vi "Pfeiffer Vacuum HiLobe Status requests.vi"(8 "error in (no error)":errorcluster, 9 "Parameter choice":T1(ring), 10 "Adress of unit":u16=1 min=1 max=999 step=1, 11 "COM Port Name in":refnum<visa-resource-name>="COM1") -> (0 "error out":errorcluster, 3 "response (data)":string)   [LabVIEW 2021]
doc: "This VI is an example of how to use the Pfeiffer Vacuum subVIs programmatically. This VI first initializes the instrument, takes measurements, then closes the instrument."
uses:
  <instrlib>/Pfeiffer Vacuum/Pfeiffer Vacuum.lvlib
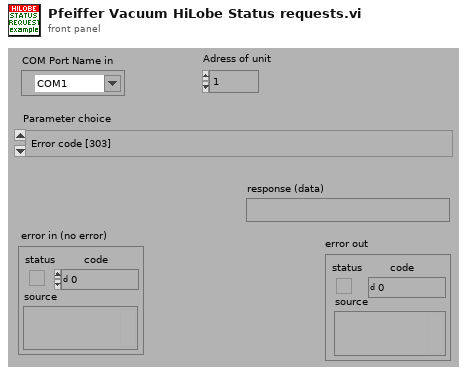
[diagram p1: front panel]
types:
  T1 = enum16{"Error code [303]", "Actual Speed (Hz) [309]", "Pump operating hours (h) [311]", "Software version of the interface board [312]", "Supply voltage (V) [313]", "Nominal speed (Hz) [315]", "Drive power (W) [316]", "Motor current (A) [317]", "Temperatur of power electronic [324]", "Device designation [349]", "Firmware of frequency converter [352]", "Hardware version of the interface board [354]", "Acutal speed (rpm) [398]", "Nominal speed (rpm) [399]"}
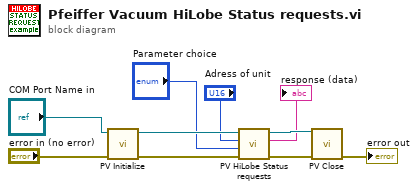
[diagram p0: block diagram]
diagram:
  n1 = call <instrlib>:"PV Initialize.vi"("error in (no error)"="error in (no error)", "VISA session in"="COM Port Name in") -> ("error out"=w10:errorcluster, "VISA session out"=w8:refnum<visa-resource-name>)  [unwired: 8 in]
  n2 = call <instrlib>:"PV HiLobe Status requests.vi"("error in (no error)"=w10, "Parameter choice"="Parameter choice", "Adress of unit"="Adress of unit", "VISA session"=w8) -> ("error out"=w9:errorcluster, "response (data)"=→"response (data)":string, "dup VISA session"=w7:refnum<visa-resource-name>)  [unwired: 5 in]
  n3 = call <instrlib>:"PV Close.vi"("VISA session"=w7, "error in (no error)"=w9) -> ("error out"=→"error out":errorcluster)  [unwired: 13 in]
